vi "pasu22.vi"() -> ()   [LabVIEW 2013]
uses:
  <vilib>/Analysis/baseanly.llb/Mean (DBL).vi
  <vilib>/Analysis/NI_AALBase.lvlib
panel:
  in  "Стоп системы":bool
  out "Данные с устройства:":string
  in  "Канал ЦАП:":i16
  out "Напряжение на фоторезисторе, В":dbl
  in  "Канал АЦП шунта:":i16
  out "Ток в цепи освещения, мА":dbl
  out "Состояние системы:":bool
  in  "Частота регистрации данных, с:":i16
  in  "Путь к log файлу:":path
  in  "Канал АЦП фоторезистора:":i16
  in  "Порог срабатывания подсветки, В":dbl
  # "Руководство пользователя\n\n1.\tПодключить плату к клеммникам питания 5В и GND контроллера (питание 5В, берется с цифрового клеммника, с клеммы под номером 19)\n2. Подключить к выводам ЦАП и АЦП на клеммнике сооветствующие выводы на плате (подключать к аналоговому клеммнику).\n3.\tУказать канал ЦАП, указать канал АЦП.\n4.\tУказать путь к *.log файлу.\n5.\tЗадать частоту регистрации данных.\n6.\tЗадать пороговое напряжение срабатывания подсветки в вольтах.\nПри достижении напряжения на фоторезисторе порогового будет включена подсветка.\n6.\tТок в цепи подсветки, напряжение на фоторезисторе, отображается на передней панели. \n7.\tДля завершение работы необходимо нажать на кнопку \"STOP\"."
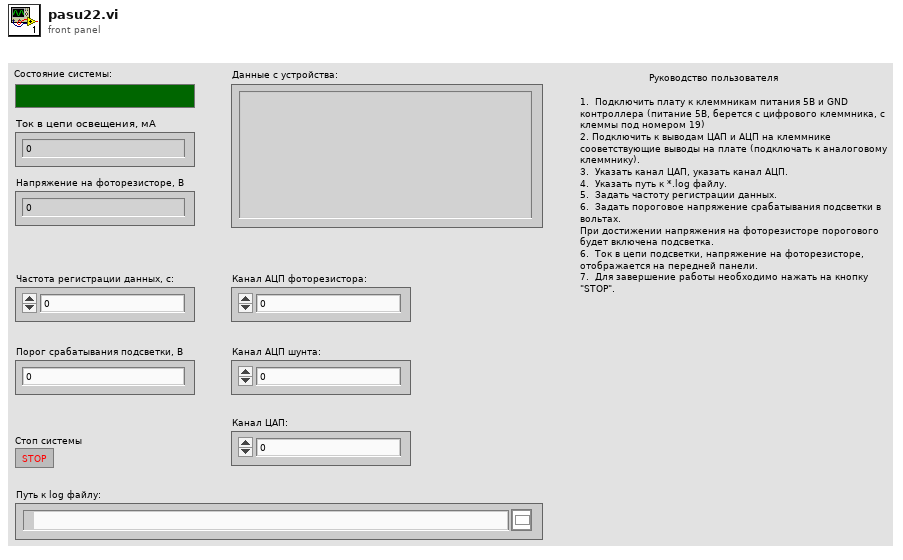
[diagram p1: front panel]
types:
  T1 = enum16{"open", "replace", "create", "open or create", "replace or create", "replace or create with confirmation"}
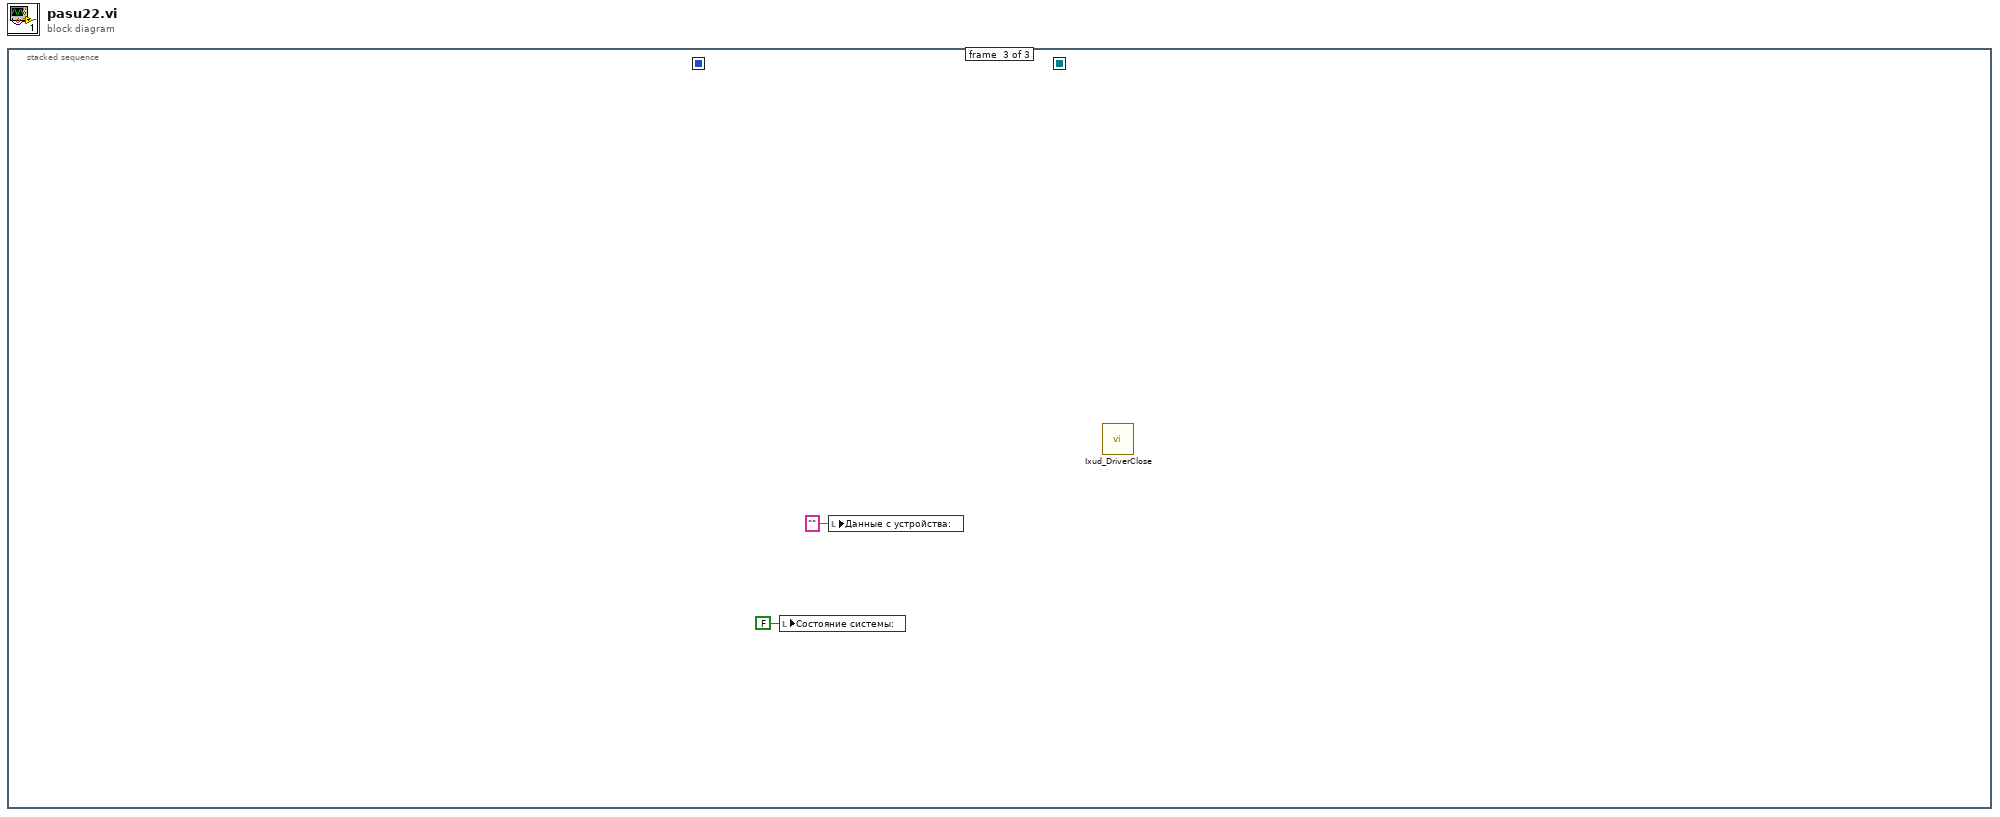
[diagram p0: block diagram]
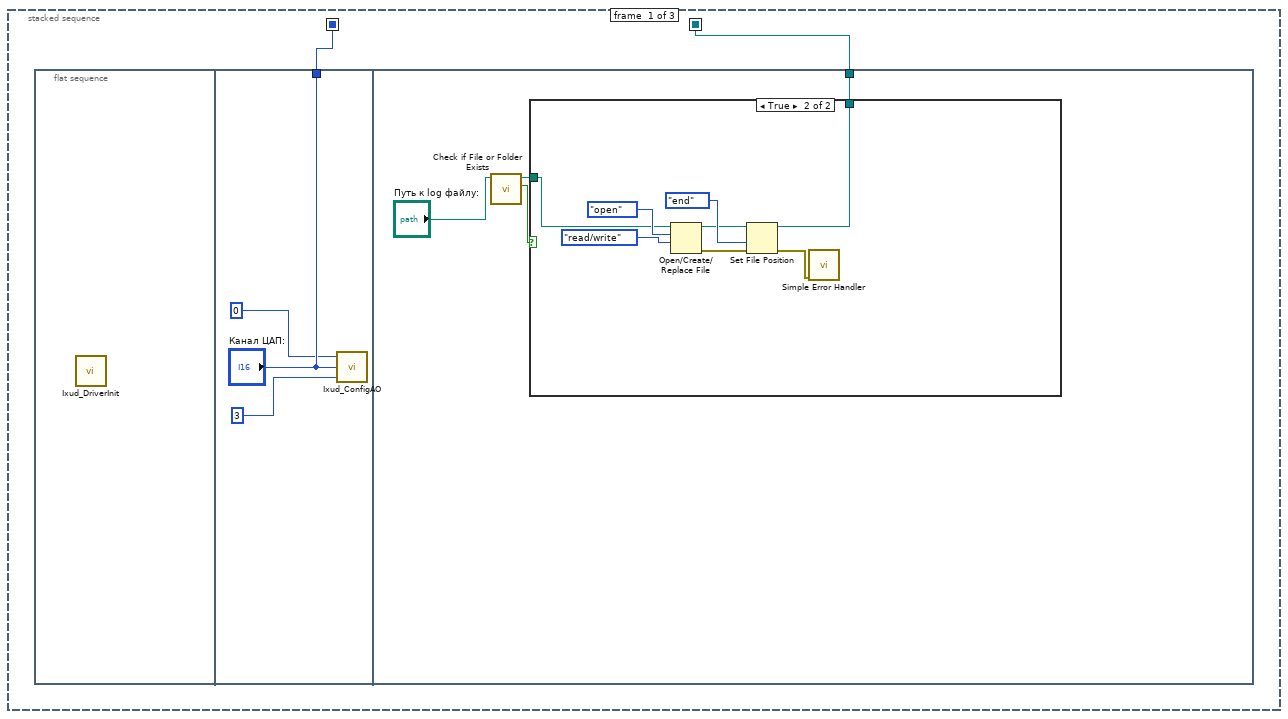
[diagram p2: hidden frame]
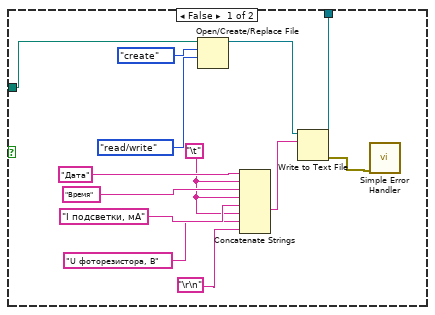
[diagram p3: hidden frame]
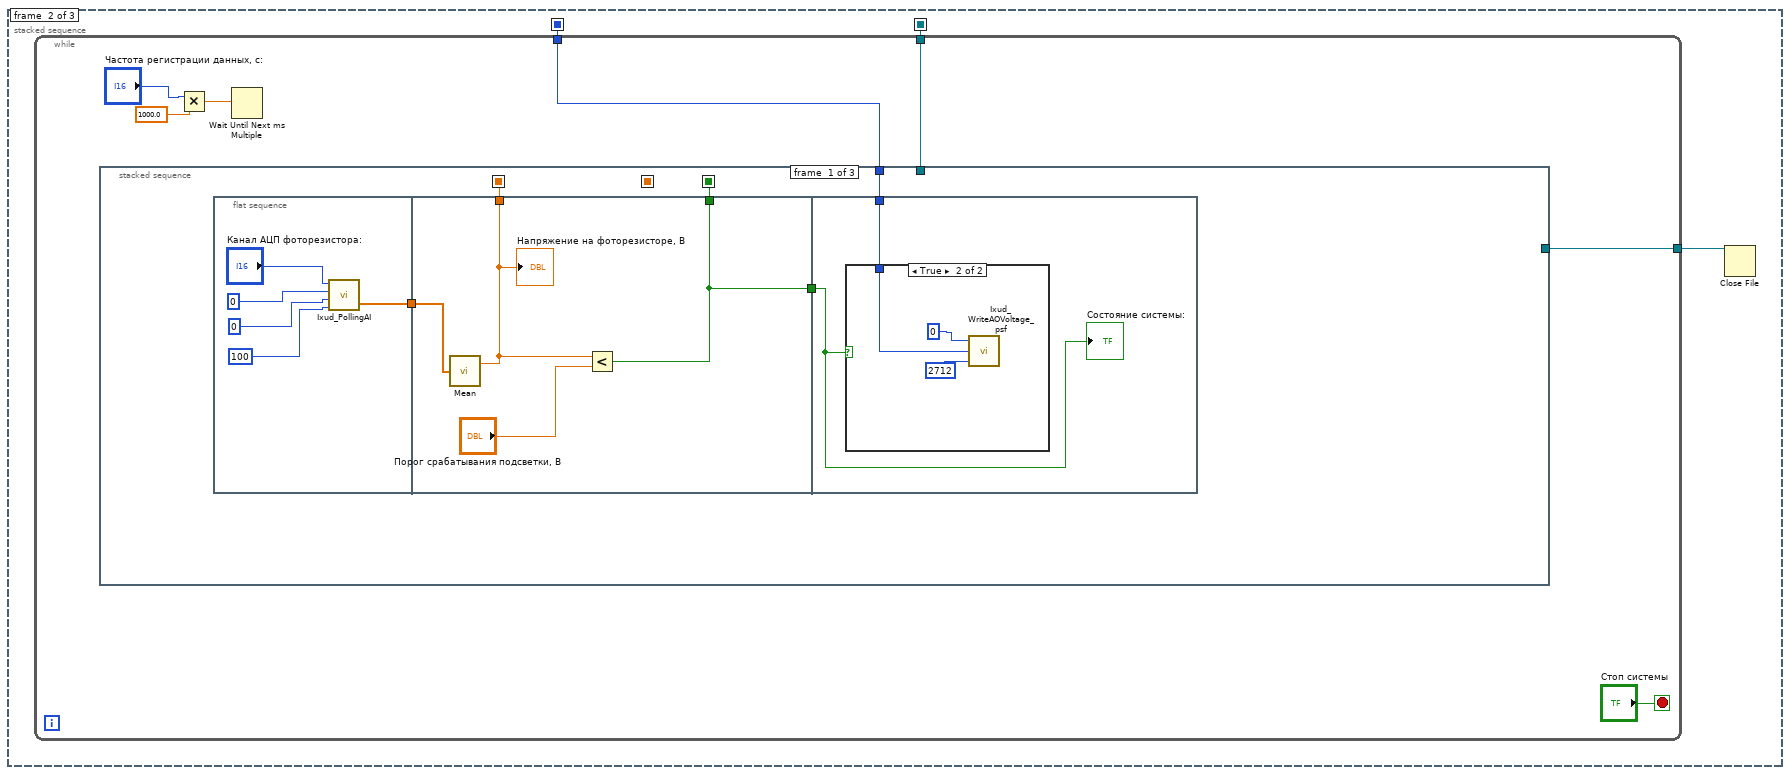
[diagram p4: hidden frame]
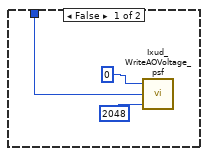
[diagram p5: hidden frame]
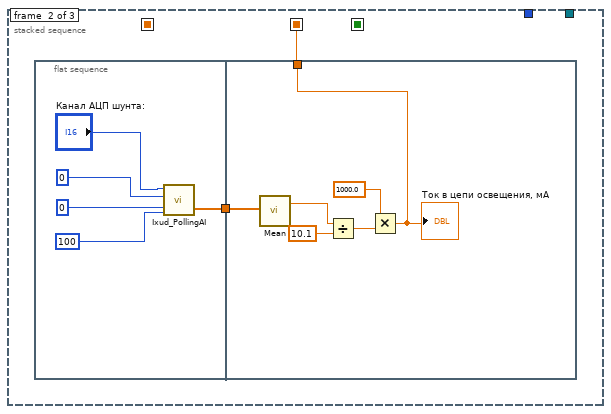
[diagram p6: hidden frame]
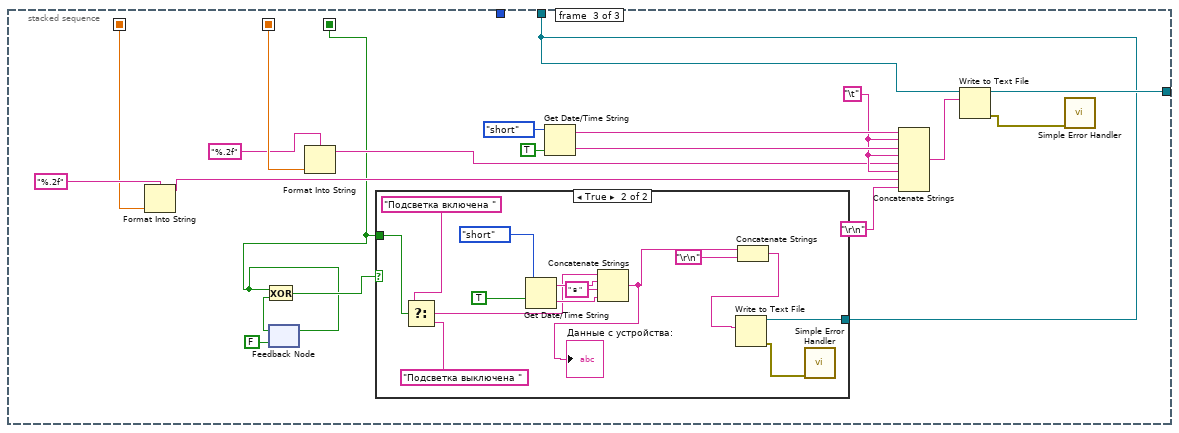
[diagram p7: hidden frame]
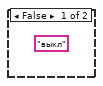
[diagram p8: hidden frame]
diagram:
  n1 = stacked-sequence {
    seq-local: [w2 _ _] -> [_ w33 _]
    seq-local: [w1 _ _] -> [_ w32 _]
    frame #0 {
      n2 = flat-sequence {
        tunnel: ["Канал ЦАП:"] -> w2
        tunnel: [w6] -> w1
        frame #0 {
          n3 = call "Ixud_DriverInit.vi"() -> ()  [unwired: 2 out]
        }
        frame #1 {
          n4 = call "Ixud_ConfigAO.vi"("wCfgCode"=3, "wChannel"="Канал ЦАП:", "wBoardNo"=0) -> ()  [unwired: 1 out]
        }
        frame #2 {
          n5 = call <vilib>:"Check if File or Folder Exists.vi"("path"="Путь к log файлу:") -> ("file or folder exists?"=w8:bool, "dup path"=w7:path)  [unwired: 8 in, 1 out]
          n6 = case shown="True" w8 {
            tunnel: w7 -> [w20 w25]
            tunnel: [w10 w24] -> w6
            frame False {
              w15 = "\t"
              n7 = Open/Create/Replace File(file path (use dialog)=w20, operation (0:open)=T1."create", access (0:read/write)=enum16{"read/write", "read-only", "write-only"}."read/write") -> (refnum out=w11:refnum<file>)  [unwired: 3 in, 2 out]
              n8 = Concatenate Strings("Дата", w15, "Время", w15, "I подсветки, мА", w15, "U фоторезистора, В", "\r\n") -> (w13:string)
              n9 = Write to Text File(file (use dialog)=w11, text=w13) -> (refnum out=w10:refnum<file>, error out=w12:errorcluster)  [unwired: 2 in, 1 out]
              n10 = call <vilib>:"Simple Error Handler.vi"("error in (no error)"=w12) -> ()  [unwired: 4 in, 5 out]
            }
            frame True {
              n11 = Open/Create/Replace File(file path (use dialog)=w25, operation (0:open)=T1."open", access (0:read/write)=enum16{"read/write", "read-only", "write-only"}."read/write") -> (refnum out=w27:refnum<file>, error out=w26:errorcluster)  [unwired: 3 in, 1 out]
              n12 = Set File Position(refnum=w27, from (0:start)=enum16{"start", "end", "current"}."end", error in=w26) -> (refnum out=w24:refnum<file>, error out=w23:errorcluster)  [unwired: 1 in]
              n13 = call <vilib>:"Simple Error Handler.vi"("error in (no error)"=w23) -> ()  [unwired: 4 in, 5 out]
            }
          }
        }
      }
    }
    frame #1 {
      n14 = while {
        tunnel: w33 -> [w39]
        tunnel: w32 -> [w35]
        tunnel: [w34] -> w31
        stop <- "Стоп системы" stop-if-true
        n15 = stacked-sequence {
          seq-local: [_ w63 _] -> [_ _ w83]
          seq-local: [w42 _ _] -> [_ _ w85]
          seq-local: [w41 _ _] -> [_ _ w76]
          tunnel: w39 -> [w44 _ _]
          tunnel: w35 -> [_ _ w78]
          tunnel: [_ _ w88] -> w34
          frame #0 {
            n16 = flat-sequence {
              tunnel: [w46] -> w45
              tunnel: w45 -> [w54]
              tunnel: [w51] -> w41
              tunnel: [w52] -> w42
              tunnel: [w51] -> w43
              tunnel: w44 -> [w56]
              tunnel: w43 -> [w55]
              frame #0 {
                n17 = call "Ixud_PollingAI.vi"("dwDataCount"=100, "wConfig"=0, "wBoardNo"=0, "wChannel"="Канал АЦП фоторезистора:") -> ("fValue"=w46:sgl[])  [unwired: 1 out]
              }
              frame #1 {
                n18 = call-poly <vilib>:"Mean.vi"("X"=w54) -> ("mean"=w52:dbl)  [unwired: 1 out]
                "Напряжение на фоторезисторе, В" <- w52
                n19 = Less?(x=w52, y="Порог срабатывания подсветки, В") -> (x < y?=w51:bool)
              }
              frame #2 {
                n20 = case shown="True" w55 {
                  tunnel: w56 -> [w57 w60]
                  frame False {
                    n21 = call "Ixud_WriteAOVoltage_psf.vi"("Code"=2048, "wChannel"=w57, "wBoardNo"=u16 0) -> ()  [unwired: 1 out]
                  }
                  frame True {
                    n22 = call "Ixud_WriteAOVoltage_psf.vi"("Code"=2712, "wChannel"=w60, "wBoardNo"=u16 0) -> ()  [unwired: 1 out]
                  }
                }
                "Состояние системы:" <- w55
              }
            }
          }
          frame #1 {
            n23 = flat-sequence {
              tunnel: [w65] -> w64
              tunnel: w64 -> [w75]
              tunnel: [w70] -> w63
              frame #0 {
                n24 = call "Ixud_PollingAI.vi"("dwDataCount"=100, "wConfig"=0, "wBoardNo"=0, "wChannel"="Канал АЦП шунта:") -> ("fValue"=w65:sgl[])  [unwired: 1 out]
              }
              frame #1 {
                n25 = call-poly <vilib>:"Mean.vi"("X"=w75) -> ("mean"=w74:dbl)  [unwired: 1 out]
                n26 = Divide(x=w74, y=10.1) -> (x/y=w72:dbl)
                n27 = Multiply(x=1000.0, y=w72) -> (x*y=w70:dbl)
                "Ток в цепи освещения, мА" <- w70
              }
            }
          }
          frame #2 {
            w91 = "\t"
            n28 = Format Into String(format string="%.2f", w85) -> (resulting string=w84:string)  [unwired: 2 in, 1 out]
            n29 = feedback #1(FALSE) -> (w80:bool)
            n30 = Exclusive Or(1:w80, 2:w76) -> (0:w77:bool)
            n31 = feedback-in #1(w76) -> ()
            n32 = Format Into String(format string="%.2f", w83) -> (resulting string=w81:string)  [unwired: 2 in, 1 out]
            n33 = case shown="True" w77 {
              tunnel: w78 -> [_ w98]
              tunnel: w76 -> [_ w96]
              frame False {
                (unwired) "выкл"
              }
              frame True {
                n34 = Select(t="Подсветка включена ", s=w96, f="Подсветка выключена ") -> (s? t:f=w102:string)
                n35 = Get Date/Time String(date format (0)=enum16{"short", "long", "abbreviated"}."short", want seconds? (F)=TRUE) -> (date string=w105:string, time string=w103:string)  [unwired: 1 in]
                n36 = Concatenate Strings(w102, w105, " в " ("string"), w103) -> (w99:string)
                "Данные с устройства:" <- w99
                n37 = Concatenate Strings(w99, "\r\n") -> (w100:string)
                n38 = Write to Text File(file (use dialog)=w98, text=w100) -> (error out=w97:errorcluster)  [unwired: 2 in, 2 out]
                n39 = call <vilib>:"Simple Error Handler.vi"("error in (no error)"=w97) -> ()  [unwired: 4 in, 5 out]
              }
            }
            n40 = Get Date/Time String(date format (0)=enum16{"short", "long", "abbreviated"}."short", want seconds? (F)=TRUE) -> (date string=w93:string, time string=w92:string)  [unwired: 1 in]
            n41 = Concatenate Strings(w93, w91, w92, w91, w81, w91, w84, "\r\n") -> (w89:string)
            n42 = Write to Text File(file (use dialog)=w78, text=w89) -> (refnum out=w88:refnum<file>, error out=w87:errorcluster)  [unwired: 2 in, 1 out]
            n43 = call <vilib>:"Simple Error Handler.vi"("error in (no error)"=w87) -> ()  [unwired: 4 in, 5 out]
          }
        }
        n44 = Multiply(x="Частота регистрации данных, с:", y=1000.0) -> (x*y=w36:dbl)
        n45 = Wait Until Next ms Multiple(millisecond multiple=w36) -> ()  [unwired: 1 out]
      }
      n46 = Close File(refnum=w31) -> ()  [unwired: 1 in, 2 out]
    }
    frame #2 {
      n47 = local write "Состояние системы:"(FALSE ("Состояние системы:")) -> ()
      n48 = local write "Данные с устройства:"("" ("Данные с устройства:")) -> ()
      n49 = call "Ixud_DriverClose.vi"() -> ()  [unwired: 1 in]
    }
  }
